vi "ziExample-Module-Scope.vi"() -> ()   [LabVIEW 2009]
doc: "Control a Zurich instrument device via the LabOne Labview API. \nRequirements: Zurich Instruments MFLI, HF2 or UHFLI \nThis example shows how to start a scope module and retrieve data.\n\n© Zurich Instruments AG, www.zhinst.com"
uses:
  <instrlib>/Zurich Instruments LabOne/Public/Modules/ziTypeModEnum.ctl
  <instrlib>/Zurich Instruments LabOne/Public/Configure/ziSetValueDouble.vi
  <instrlib>/Zurich Instruments LabOne/Public/Modules/ziModSetValueDoubleArray.vi
  <instrlib>/Zurich Instruments LabOne/Public/Configure/ziGetValueString.vi
  <instrlib>/Zurich Instruments LabOne/Public/Configure/ziSetValueDoubleArray.vi
  <instrlib>/Zurich Instruments LabOne/Public/Modules/ziModGetScopeWave.vi
  <instrlib>/Zurich Instruments LabOne/Public/Modules/ziModSetValueDouble.vi
  <instrlib>/Zurich Instruments LabOne/Zurich Instruments LabOne.lvlib
panel:
  in  "length":i32=100 caption="Length (pts)"
  in  "segmentedcount":i32=100 caption="segmented count"
  in  "segmented":bool=TRUE
  out "?":sgl[][](graph)
  in  "mode":u16(ring)=1 items=["Time Domain"=1, "Freq Domain FFT"=3]
  in  "stop":bool
  in  "averagerweight":dbl=1.0 caption="averager/weight"
  out "?":cluster{dbl[], "Data Float":sgl[]}[](graph)
  out "Error Out":errorcluster
  in  "Address":string="DEV"
  out "Selected Device":string
  in  "subscribepath":string="scopes/0/wave" caption="Subscribe Path"
  # "Only for non-HF2"
  # "ziExample-SweepModul.vi\nRequirements: HF2LI, UHFLI or MFLI\nsee block diagram for VI description"
  # "Tested Devices:\n- HF2LI\n- UHFLI\n- MFLI"
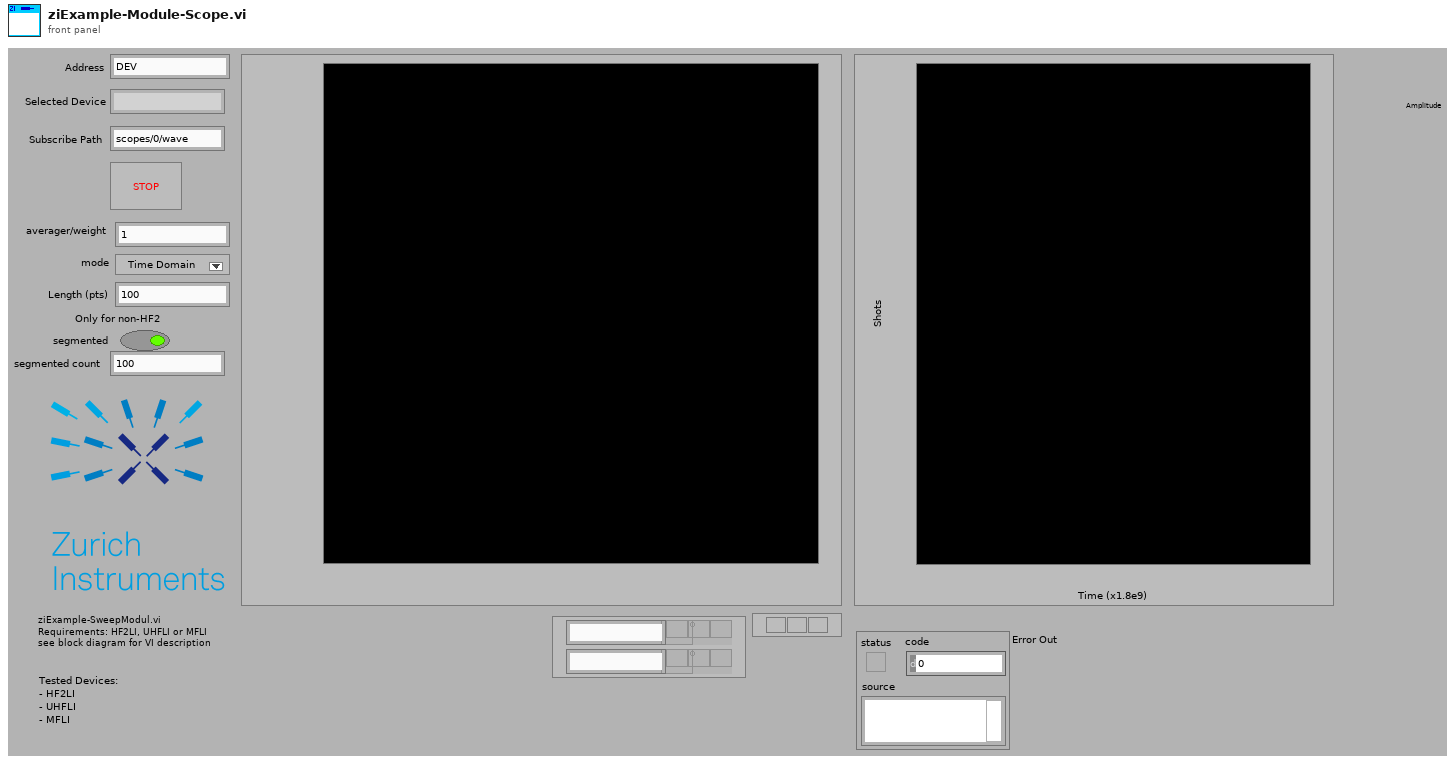
[diagram p1: front panel]
types:
  T1 = typedef "Zurich Instruments LabOne.lvlib/ziTypeModEnum.ctl" = u16
  T2 = typedef "Zurich Instruments LabOne.lvlib/ziTypeHandle.ctl" = cluster{"handleValid":bool, "Conn":u64, "Path Prefix":string, "Handle":u64, "Connected":bool, "Clockbase(s)":dbl}
  T3 = typedef "Zurich Instruments LabOne.lvlib/ziTypeModHandle.ctl" = cluster{"handleValid":bool, "Conn":u64, "ModHandle":u64, "moduleID":string, "Path Prefix":string}
  T4 = typedef "Zurich Instruments LabOne.lvlib/ziTypeModResults.ctl" = cluster{"PathArray":string[], "ValueType":T5, "NoOfResults":u64, "ziGenericHeader":T6[]}
  T5 = typedef "Zurich Instruments LabOne.lvlib/ziTypePollType.ctl" = enum16{"NONE", "DOUBLE_DATA", "INTEGER_DATA", "DEMOD_SAMPLE", "SCOPE_WAVE_HF2", "AUXIN_SAMPLE", "DIO_SAMPLE", "BYTE_ARRAY", "PWA_WAVE", "9", "10", "11", "12", "13", "14", "15", "TREE_CHANGE_DEPRI", "17", "ERROR", "19", "20", "21", "22", "23", "24", "25", "26", "27", "28", "29", "30", "31", "DOUBLE_DATA_TS", "INTEGER_DATA_TS", "34", "SCOPE_WAVE", "SCOPE_WAVE_EX", "37", "BYTE_ARRAY_TS", "39", "40", "41", "42", "43", "44", "45", "CNT_DATA", "47", "TREE_CHANGE", "49", "50", "51", "52", "53", "54", "55", "56", "57", "58", "59", "60", "61", "62", "63", "SWEEPER_DATA", "SPECTRUM_DATA", "ADVISOR_DATA", "VECTOR_DATA", "IMP_DATA"}
  T6 = typedef "Zurich Instruments LabOne.lvlib/ziTypeModGenericHeader.ctl" = cluster{"HeaderType":enum8{"HEADER_TYPE_NONE", "HEADER_TYPE_SWTRIGGER", "HEADER_TYPE_SWEEPER"}, "SampleFormat":u8, "SystemTime":timestamp, "CreatedTimeStamp":u64, "ChangedTimeStamp":u64, "Flags":u32, "ChunkSizeBytes":u64, "Name":string, "Status":u32, "GroupIndex":u32, "Color":u32, "ActiveRow":u32, "TriggerNumber":u64, "GridRows":u32, "GridCols":u32, "GridMode":u32, "GridOperation":u32, "GridDirection":u32, "GridRepetitions":u32, "GridColDelta":dbl, "GridColOffset":dbl, "GridRowDelta":dbl, "GridRowOffset":dbl, "Bandwidth":dbl, "Center":dbl, "Nenbw":dbl}
  T7 = typedef "Zurich Instruments LabOne.lvlib/ziTypeScopeWaveGrid.ctl" = cluster{"Timestamp (ticks)":u64, "Timestamp Trigger (ticks)":u64, "dt (s)":dbl, "Channel Enable":u8[], "Channel Input":enum8{"Signal Input 1", "Signal Input 2", "Trigger Input 1", "Trigger Input 2", "Aux Output 1", "Aux Output 2", "Aux Output 3", "Aux Output 4", "Aux Input 1", "Aux Input 2"}[], "Trigger Enable":u64, "Trigger Input":u64, "Channel BW Limit":u8[], "Channel Math":u8[], "Channel Scaling":sgl[], "Sequence Number":u32, "Segment Number":u32, "Block Number":u32, "Data Transfer Mode":enum8{"Single Transfer", "Block Transfer", "Continuous Transfer", "FFT Single Transfer"}, "Block Marker":enum8{"None", "End of Block"}, "Flags":u8, "Sample Format":enum8{"Int16", "Int32", "Float32", "reserved", "Int16 Interleaved", "Int32 Interleaved", "Float32 Interleaved"}, "Sample Count":u32, "Channel Offset":dbl[], "Data Int16":i16[][], "Data Int32":i32[][], "Data Float":sgl[][], "Total Samples":u32}
  T8 = typedef "Zurich Instruments LabOne.lvlib/ziTypeScopeWave.ctl" = cluster{"Timestamp (ticks)":u64, "Timestamp Trigger (ticks)":u64, "dt (s)":dbl, "Channel Enable":u8[], "Channel Input":enum8{"Signal Input 1", "Signal Input 2", "Trigger Input 1", "Trigger Input 2", "Aux Output 1", "Aux Output 2", "Aux Output 3", "Aux Output 4", "Aux Input 1", "Aux Input 2"}[], "Trigger Enable":u64, "Trigger Input":u64, "Channel BW Limit":u8[], "Channel Math":u8[], "Channel Scaling":sgl[], "Sequence Number":u32, "Segment Number":u32, "Block Number":u32, "Data Transfer Mode":enum8{"Single Transfer", "Block Transfer", "Continuous Transfer", "FFT Single Transfer"}, "Block Marker":enum8{"None", "End of Block"}, "Flags":u8, "Sample Format":enum8{"Int16", "Int32", "Float32", "reserved", "Int16 Interleaved", "Int32 Interleaved", "Float32 Interleaved"}, "Sample Count":u32, "Channel Offset":dbl[], "Data Int16":i16[], "Data Int32":i32[], "Data Float":sgl[], "Total Samples":u64}
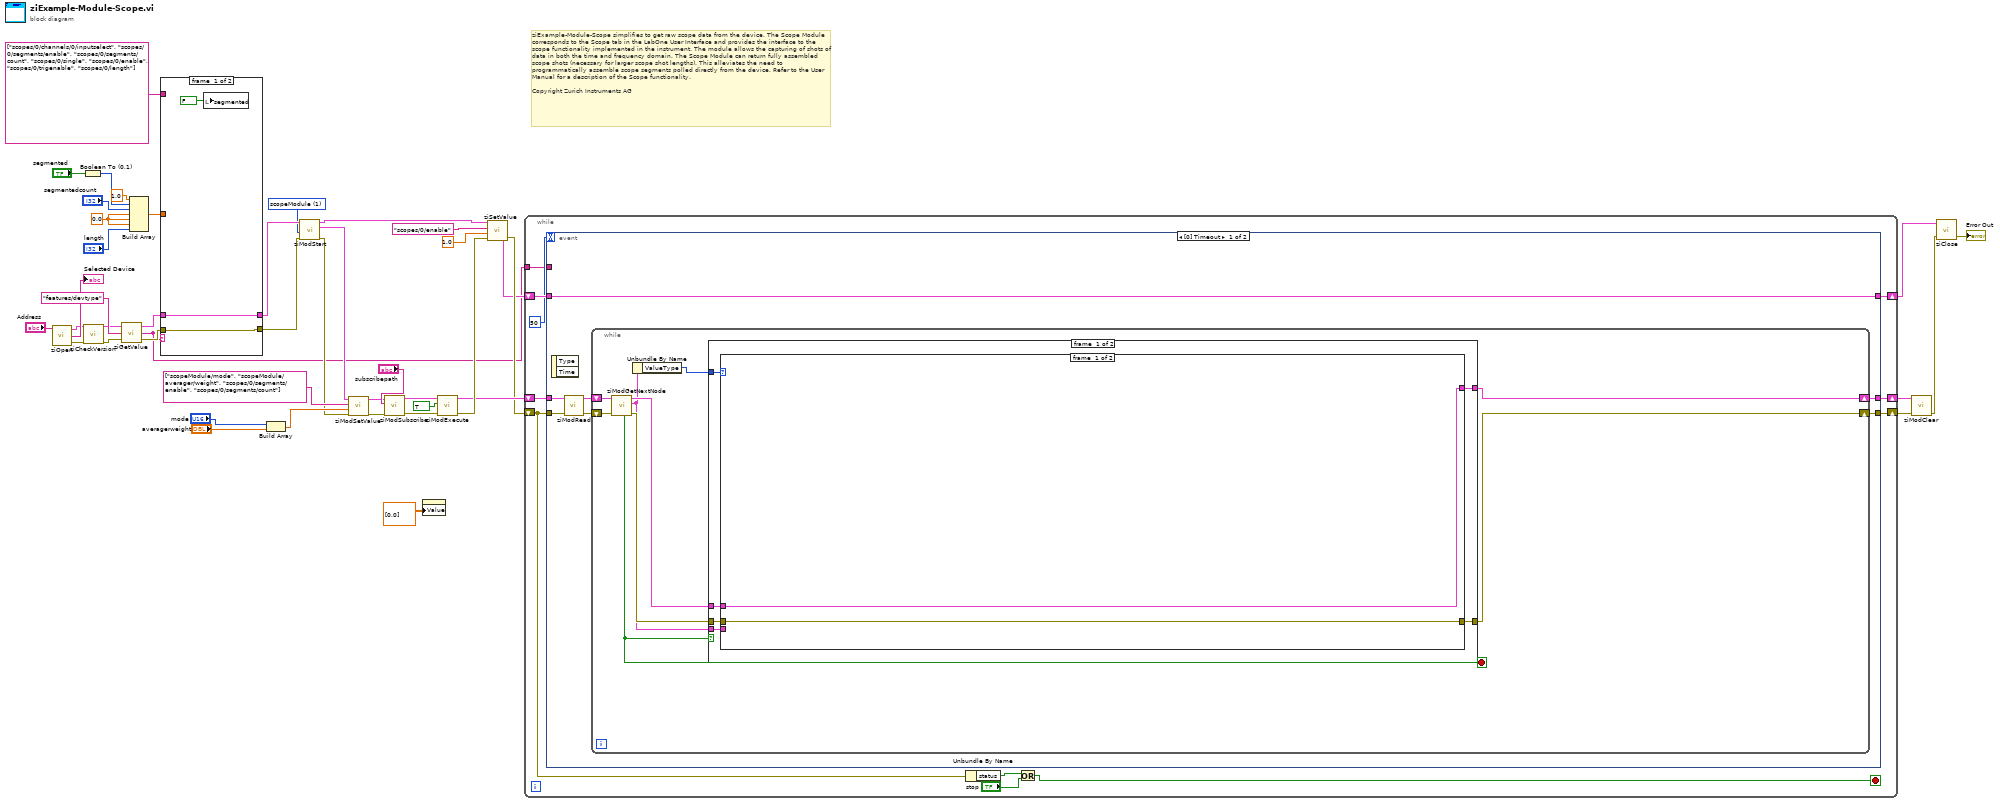
[diagram p0: block diagram]
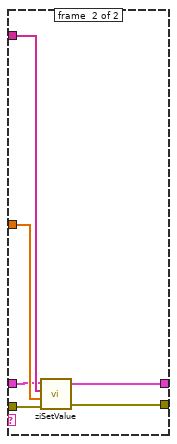
[diagram p2: hidden frame]
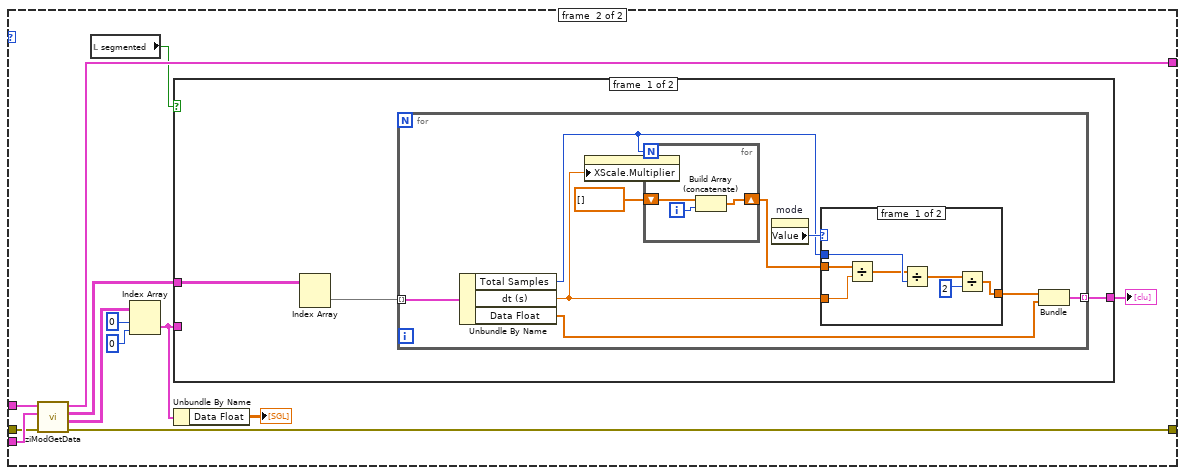
[diagram p3: hidden frame]
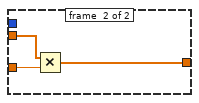
[diagram p4: hidden frame]
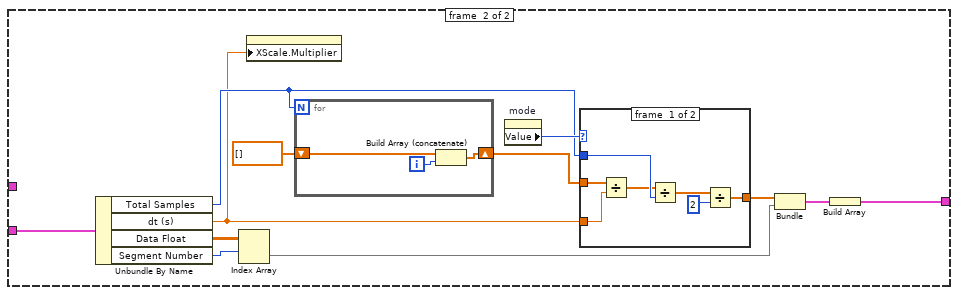
[diagram p5: hidden frame]
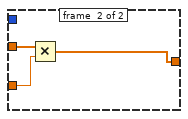
[diagram p6: hidden frame]
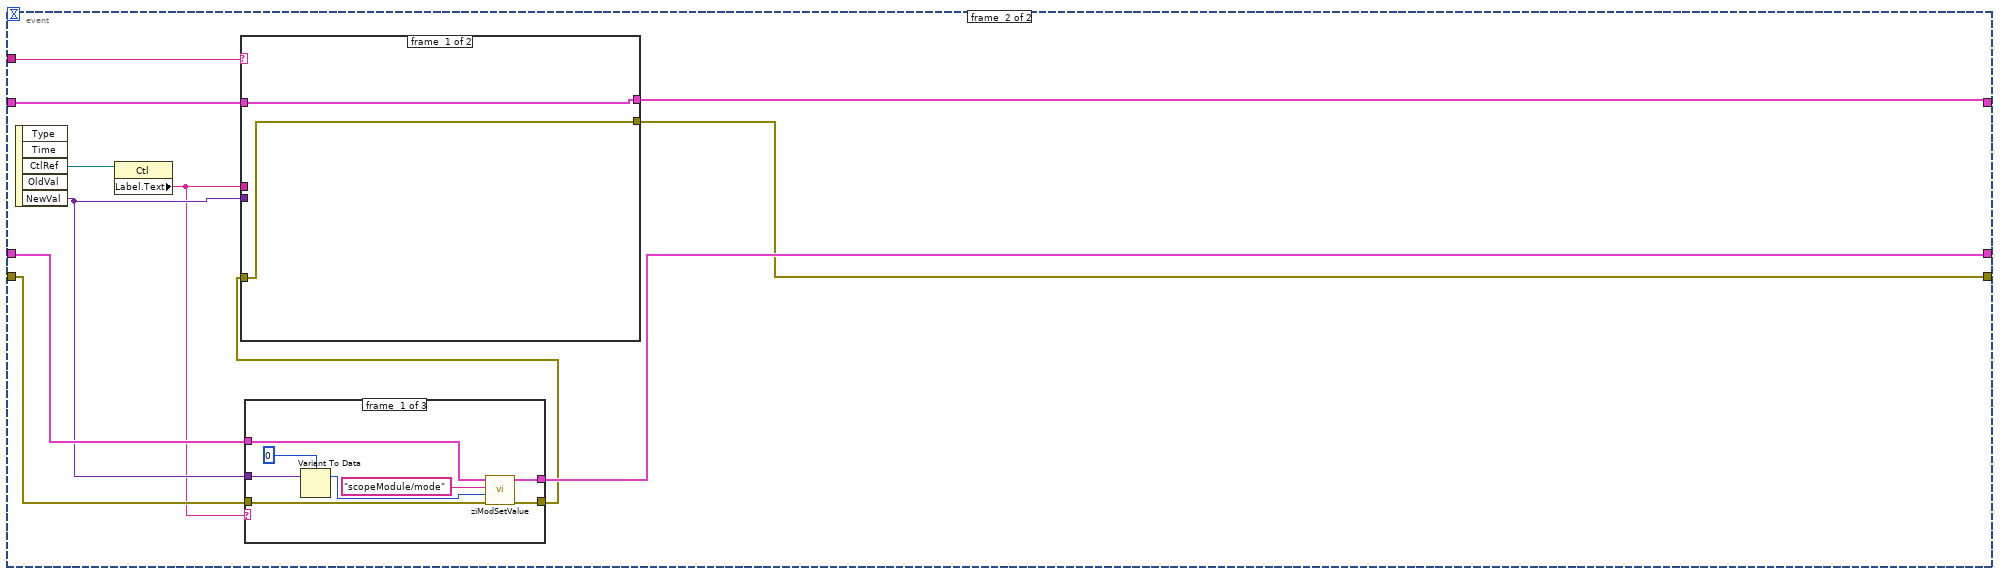
[diagram p8: hidden frame]
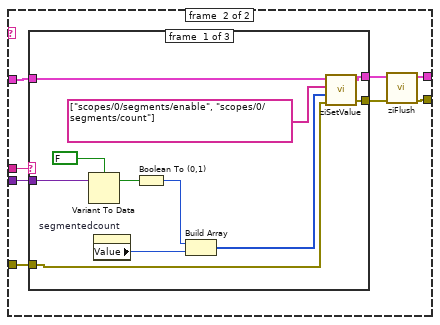
[diagram p9: hidden frame]
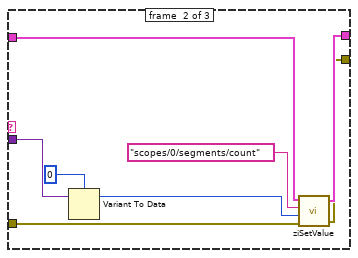
[diagram p10: hidden frame]
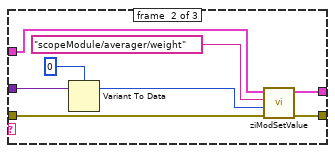
[diagram p12: hidden frame]
diagram:
  w3 = T1 1 items=["sweep", "scopeModule", "dataAcquisitionModule", "pidAdvisor", "awgModule", "impedanceModule", "multiDeviceSyncModule", "zoomFFT", "trigger", "deviceSettings", "record"] ("module Id")
  w9 = 0.0 ("element")
  # "ziExample-Module-Scope simplifies to get raw scope data from the device. The Scope Module corresponds to the Scope tab in the LabOne User Interface and provides the interface to the scope functionality implemented in the instrument. The module allows the capturing of shots of data in both the time and frequency domain. The Scope Module can return fully assembled scope shots (necessary for larger scope shot lengths). This alleviates the need to programmatically assemble scope segments polled directly from the device. Refer to the User Manual for a description of the Scope functionality.\n\nCopyright Zurich Instruments AG"
  n1 = call <instrlib>:"ziOpen.vi"("Address"="Address") -> ("Error Out"=w6:errorcluster, "Selected Device"=→"Selected Device":string, "HandleOut"=w7:T2)  [unwired: 1 in, 2 out]
  n2 = Boolean To (0,1)(Boolean="segmented") -> (0, 1=w24:i16)
  n3 = call <instrlib>:"ziCheckVersion.vi"("Handle In"=w7, "Error In"=w6) -> ("Handle Out"=w4:T2, "Error Out"=w5:errorcluster)  [unwired: 11 in, 1 out]
  n4 = call-poly <instrlib>:"ziGetValue.vi"("error in"=w5, "Path"="features/devtype", "Handle In"=w4) -> ("error out"=w12:errorcluster, "Value"=w11:string, "Handle Out"=w13:T2)
  n5 = Build Array(1.0 ("element"), w24, "segmentedcount", w9, w9, w9, "length") -> (w26:dbl[])
  n6 = case shown="\"HF2IS\", \"HF2LI\"" w11 {
    tunnel: [w48 w55] -> w44
    tunnel: string[] ["scopes/0/channels/0/inputselect", "scopes/0/segments/enable", "scopes/0/segments/count", "scopes/0/single", "scopes/0/enable", "scopes/0/trigenable", "scopes/0/length"] -> [_ w54]
    tunnel: [w49 w53] -> w31
    tunnel: w26 -> [_ w52]
    tunnel: w13 -> [w49 w51]
    tunnel: w12 -> [w48 w50]
    frame #0 {
      n7 = local write "segmented"(FALSE ("segmented")) -> ()
    }
    frame #1 {
      n8 = call-poly <instrlib>:"ziSetValue.vi"("Error In"=w50, "Values"=w52, "Paths"=w54, "Handle In"=w51) -> ("Error Out"=w55:errorcluster, "Handle Out"=w53:T2)  [unwired: 1 in]
    }
  }
  n9 = Build Array("mode", "averagerweight") -> (w22:dbl[])
  n10 = call <instrlib>:"ziModStart.vi"("Error In"=w44, "module Id"=w3, "Handle In"=w31) -> ("Error Out"=w17:errorcluster, "ModHandle Out"=w18:T3, "Handle Out"=w10:T2)  [unwired: 6 in]
  n11 = call-poly <instrlib>:"ziModSetValue.vi"("Error In"=w17, "Values"=w22, "Paths"=string[] ["scopeModule/mode", "scopeModule/averager/weight", "scopes/0/segments/enable", "scopes/0/segments/count"], "ModHandle In"=w18) -> ("Error Out"=w16:errorcluster, "ModHandle Out"=w15:T3)  [unwired: 6 in]
  n12 = call <instrlib>:"ziModSubscribe.vi"("Error In"=w16, "Path"="subscribepath", "ModHandle In"=w15) -> ("Error Out"=w36:errorcluster, "ModHandle Out"=w37:T3)  [unwired: 6 in]
  n13 = property class="IntGraph (strict)"("Value"=dbl[][] [[0.0]]) -> ()  [unwired: 2 in, 2 out]
  n14 = call <instrlib>:"ziModExecute.vi"("Error In"=w36, "Modal (F)"=TRUE ("Modal"), "ziModHandle In"=w37) -> ("Error Out"=w35:errorcluster, "ziModHandle Out"=w30:T3)  [unwired: 5 in, 1 out]
  n15 = call-poly <instrlib>:"ziSetValue.vi"("Error In"=w35, "Value"=1.0, "Path"="scopes/0/enable", "Handle In"=w10) -> ("Error Out"=w29:errorcluster, "Handle Out"=w28:T2)  [unwired: 1 in]
  n16 = while {
    shift-right: [w65] -> w41
    shift-left: w29 -> [w56]
    shift-right: [w64] -> w40
    shift-left: w30 -> [w66]
    shift-right: [w62] -> w27
    shift-left: w28 -> [w63]
    tunnel: w11 -> [w60]
    stop <- w57 stop-if-true
    n17 = event shown="[0] Timeout" {
      selector: _ -> [_ _]
      dyn-events: _ -> [_ _]
      timeout: 50 -> [_ _]
      tunnel: w66 -> [w71 w164]
      tunnel: w56 -> [w70 w165]
      tunnel: [w69 w161] -> w65
      tunnel: [w68 w163] -> w64
      tunnel: w63 -> [w67 w160]
      tunnel: [w67 w162] -> w62
      tunnel: w60 -> [_ w156]
      event #0 {
        n18 = event-data() -> ()  [unwired: 1 in, 2 out]
        n19 = call <instrlib>:"ziModRead.vi"("error in"=w70, "ziModHandle In"=w71) -> ("error out"=w73:errorcluster, "ziModHandle Out"=w72:T3)  [unwired: 8 in]
        n20 = while {
          shift-right: [w81] -> w68
          shift-left: w72 -> [w75]
          shift-right: [w80] -> w69
          shift-left: w73 -> [w76]
          stop <- w74 stop-if-true
          n21 = call <instrlib>:"ziModGetNextNode.vi"("Error In"=w76, "ModHandle In"=w75) -> ("Error Out"=w79:errorcluster, "ModResults"=w77:T4, "ModHandle Out"=w82:T3, "NoData"=w74:bool)  [unwired: 6 in]
          n22 = Unbundle By Name(w77) -> ("ValueType"=w78:T5)
          n23 = case shown="False" w74 {
            tunnel: w82 -> [w88 w154]
            tunnel: [w87 w154] -> w81
            tunnel: [w86 w155] -> w80
            tunnel: w79 -> [w85 w155]
            tunnel: w77 -> [w84 _]
            tunnel: w78 -> [w83 _]
            frame #0 {
              n24 = case shown="\"SCOPE_WAVE_EX\"" w83 {
                tunnel: w88 -> [w90 w100]
                tunnel: w84 -> [_ w103]
                tunnel: w85 -> [w89 w102]
                tunnel: [w89 w101] -> w86
                tunnel: [w90 w99] -> w87
                frame #0 {
                }
                frame #1 {
                  n25 = call-poly <instrlib>:"ziModGetData.vi"("Error In"=w102, "ModResults"=w103, "ModHandle In"=w100) -> ("Error Out"=w101:errorcluster, "ModScopeWaveGrid"=w97:T7[][], "ModScopeWave"=w93:T8[][], "ModHandle Out"=w99:T3)  [unwired: 5 in]
                  n26 = local read "segmented"() -> (w92:bool)
                  n27 = Index Array(array=w97, index (row)=0, index (col)=0 ("disabled index (col)")) -> (element=w91:T7)
                  n28 = case shown="True" w92 {
                    tunnel: [w106 w131] -> w98
                    tunnel: w93 -> [w105 _]
                    tunnel: w91 -> [_ w140]
                    frame #0 {
                      n29 = Index Array(array=w105) -> (element=w104:T8[])  [unwired: 2 in]
                      n30 = for {
                        tunnel: w104 -> [w115] mode=indexing
                        tunnel: [w113] -> w106 mode=indexing
                        n31 = Unbundle By Name(w115) -> ("Total Samples"=w109:u64, "dt (s)"=w107:dbl, "Data Float"=w112:sgl[])
                        n32 = property class="IntGraph (strict)"("XScale.Multiplier"=w107) -> ()  [unwired: 2 in, 2 out]
                        n33 = for {
                          N: w109 -> [_]
                          shift-right: [w127] -> w110
                          shift-left: dbl[] [] -> [w128]
                          i -> [w126]
                          n34 = Build Array (concatenate)(w128, w126) -> (w127:dbl[])
                        }
                        n35 = property on="mode" class="Ring (strict)"() -> ("Value"=w111:u16)  [unwired: 2 in, 2 out]
                        n36 = case shown="1, Default" w111 {
                          tunnel: w107 -> [w122 w125]
                          tunnel: w110 -> [w121 w124]
                          tunnel: w109 -> [w120 _]
                          tunnel: [w116 w123] -> w108
                          frame #0 {
                            n37 = Divide(x=w121, y=w122) -> (x/y=w119:dbl[])
                            n38 = Divide(x=w119, y=w120) -> (x/y=w118:dbl[])
                            n39 = Divide(x=w118, y=2) -> (x/y=w116:dbl[])
                          }
                          frame #1 {
                            n40 = Multiply(x=w124, y=w125) -> (x*y=w123:dbl[])
                          }
                        }
                        n41 = Bundle(w108, "Data Float"=w112) -> (w113:cluster{dbl[], "Data Float":sgl[]})  [unwired: 1 in]
                      }
                    }
                    frame #1 {
                      n42 = Unbundle By Name(w140) -> ("Total Samples"=w136:u32, "dt (s)"=w134:dbl, "Data Float"=w130:sgl[][], "Segment Number"=w129:u32)
                      n43 = Index Array(array=w130, index (row)=w129) -> (element=w133:sgl[])  [unwired: 1 in]
                      n44 = property class="IntGraph (strict)"("XScale.Multiplier"=w134) -> ()  [unwired: 2 in, 2 out]
                      n45 = for {
                        N: w136 -> [_]
                        shift-right: [w152] -> w137
                        shift-left: dbl[] [] -> [w153]
                        i -> [w151]
                        n46 = Build Array (concatenate)(w153, w151) -> (w152:dbl[])
                      }
                      n47 = property on="mode" class="Ring (strict)"() -> ("Value"=w138:u16)  [unwired: 2 in, 2 out]
                      n48 = case shown="1, Default" w138 {
                        tunnel: w134 -> [w147 w150]
                        tunnel: w137 -> [w146 w149]
                        tunnel: w136 -> [w145 _]
                        tunnel: [w141 w148] -> w135
                        frame #0 {
                          n49 = Divide(x=w146, y=w147) -> (x/y=w144:dbl[])
                          n50 = Divide(x=w144, y=w145) -> (x/y=w143:dbl[])
                          n51 = Divide(x=w143, y=2) -> (x/y=w141:dbl[])
                        }
                        frame #1 {
                          n52 = Multiply(x=w149, y=w150) -> (x*y=w148:dbl[])
                        }
                      }
                      n53 = Bundle(w135, "Data Float"=w133) -> (w132:cluster{dbl[], "Data Float":sgl[]})  [unwired: 1 in]
                      n54 = Build Array(w132) -> (w131:cluster{dbl[], "Data Float":sgl[]}[])
                    }
                  }
                  "?" <- w98
                  n55 = Unbundle By Name(w91) -> ("Data Float"=→"?":sgl[][])
                }
              }
            }
            frame #1 {
            }
          }
        }
      }
      event #1 {
        n56 = event-data() -> ("CtlRef"=w166:refnum<vi>, "NewVal"=w158:variant)  [unwired: 1 in, 3 out]
        n57 = property class="Ctl"(reference=w166) -> ("Label.Text"=w157:string)  [unwired: 1 in, 2 out]
        n58 = case shown="\"mode\"" w157 {
          tunnel: w158 -> [w205 w213 _]
          tunnel: w165 -> [w202 w210 w215]
          tunnel: [w201 w209 w215] -> w159
          tunnel: w164 -> [w200 w208 w214]
          tunnel: [w199 w207 w214] -> w163
          frame #0 {
            n59 = Variant To Data(Variant=w205, type=u16 0) -> (data=w203:u16)  [unwired: 1 in, 1 out]
            n60 = call-poly <instrlib>:"ziModSetValue.vi"("Error In"=w202, "Value"=w203, "Path"="scopeModule/mode", "ModHandle In"=w200) -> ("Error Out"=w201:errorcluster, "ModHandle Out"=w199:T3)  [unwired: 6 in]
          }
          frame #1 {
            n61 = Variant To Data(Variant=w213, type=0) -> (data=w211:i32)  [unwired: 1 in, 1 out]
            n62 = call-poly <instrlib>:"ziModSetValue.vi"("Error In"=w210, "Value"=w211, "Path"="scopeModule/averager/weight", "ModHandle In"=w208) -> ("Error Out"=w209:errorcluster, "ModHandle Out"=w207:T3)  [unwired: 6 in]
          }
          frame #2 {
          }
        }
        n63 = case shown="Default" w156 {
          tunnel: [w167 w176] -> w162
          tunnel: [w168 w175] -> w161
          tunnel: w160 -> [w167 w173]
          tunnel: w159 -> [w168 w172]
          tunnel: w158 -> [_ w171]
          tunnel: w157 -> [_ w170]
          frame #0 {
          }
          frame #1 {
            n64 = case shown="\"segmented\"" w170 {
              tunnel: w171 -> [w187 w195 _]
              tunnel: w173 -> [w184 w192 w197]
              tunnel: [w183 w191 w197] -> w174
              tunnel: w172 -> [w182 w190 w196]
              tunnel: [w181 w189 w196] -> w169
              frame #0 {
                n65 = Variant To Data(Variant=w187, type=FALSE ("segmented 2")) -> (data=w185:bool)  [unwired: 1 in, 1 out]
                n66 = property on="segmentedcount" class="DigNum (strict)"() -> ("Value"=w177:i32)  [unwired: 2 in, 2 out]
                n67 = Boolean To (0,1)(Boolean=w185) -> (0, 1=w179:i16)
                n68 = Build Array(w179, w177) -> (w178:i32[])
                n69 = call-poly <instrlib>:"ziSetValue.vi"("Error In"=w182, "Values"=w178, "Paths"=string[] ["scopes/0/segments/enable", "scopes/0/segments/count"], "Handle In"=w184) -> ("Error Out"=w181:errorcluster, "Handle Out"=w183:T2)  [unwired: 1 in]
              }
              frame #1 {
                n70 = Variant To Data(Variant=w195, type=0) -> (data=w194:i32)  [unwired: 1 in, 1 out]
                n71 = call-poly <instrlib>:"ziSetValue.vi"("Error In"=w190, "Value"=w194, "Path"="scopes/0/segments/count", "Handle In"=w192) -> ("Error Out"=w189:errorcluster, "Handle Out"=w191:T2)  [unwired: 1 in]
              }
              frame #2 {
              }
            }
            n72 = call <instrlib>:"ziFlush.vi"("error in"=w169, "Handle In"=w174) -> ("error out"=w175:errorcluster, "Handle Out"=w176:T2)  [unwired: 8 in]
          }
        }
      }
    }
    n73 = Unbundle By Name(w56) -> ("status"=w59:bool)
    n74 = Or(x=w59, y="stop") -> (x .or. y?=w57:bool)
  }
  n75 = call <instrlib>:"ziModClear.vi"("Error In"=w41, "ziModHandle In"=w40) -> ("Error Out"=w46:errorcluster)  [unwired: 7 in, 1 out]
  n76 = call <instrlib>:"ziClose.vi"("Error In"=w46, "Handle In"=w27) -> ("Error Out"=→"Error Out":errorcluster)  [unwired: 2 in, 1 out]
